vi "Test.vi"() -> ()   [LabVIEW 2015, in "Database.lvclass"]
uses:
  Database.lvclass
  <vilib>/addons/database/Auxilliary.llb/DB Tools Column Info.ctl
  <vilib>/addons/database/Auxilliary.llb/DB Tools DataTypes.ctl
  <vilib>/addons/database/NI_Database_API.lvlib
panel:
  out "Not Empty":bool
  out "eof?":bool
  in  "data":T1
  in  "columns":string[](array[string])
  out "recordset data":variant[][](array[variant])
  in  "condition":string
  in  "column information":T2[](array[typedef])
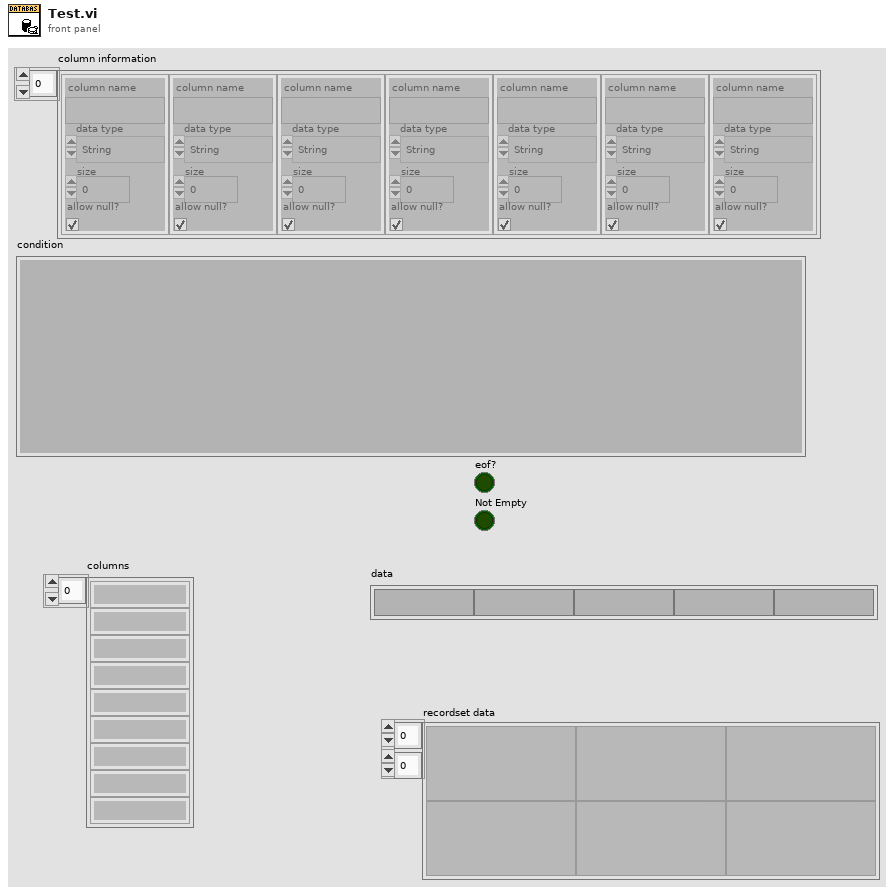
[diagram p1: front panel]
types:
  T1 = cluster{"String":string, "String 2":string, "String 3":string, "String 4":string, "String 5":string}
  T2 = typedef "NI_Database_API.lvlib/DB Tools Column Info.ctl" = cluster{"column name":string, "data type":T3, "size":i32, "allow null?":bool}
  T3 = typedef "NI_Database_API.lvlib/DB Tools DataTypes.ctl" = enum16{"String", "Long (I32)", "Single (SGL)", "Double (DBL)", "Date/Time", "Binary"}
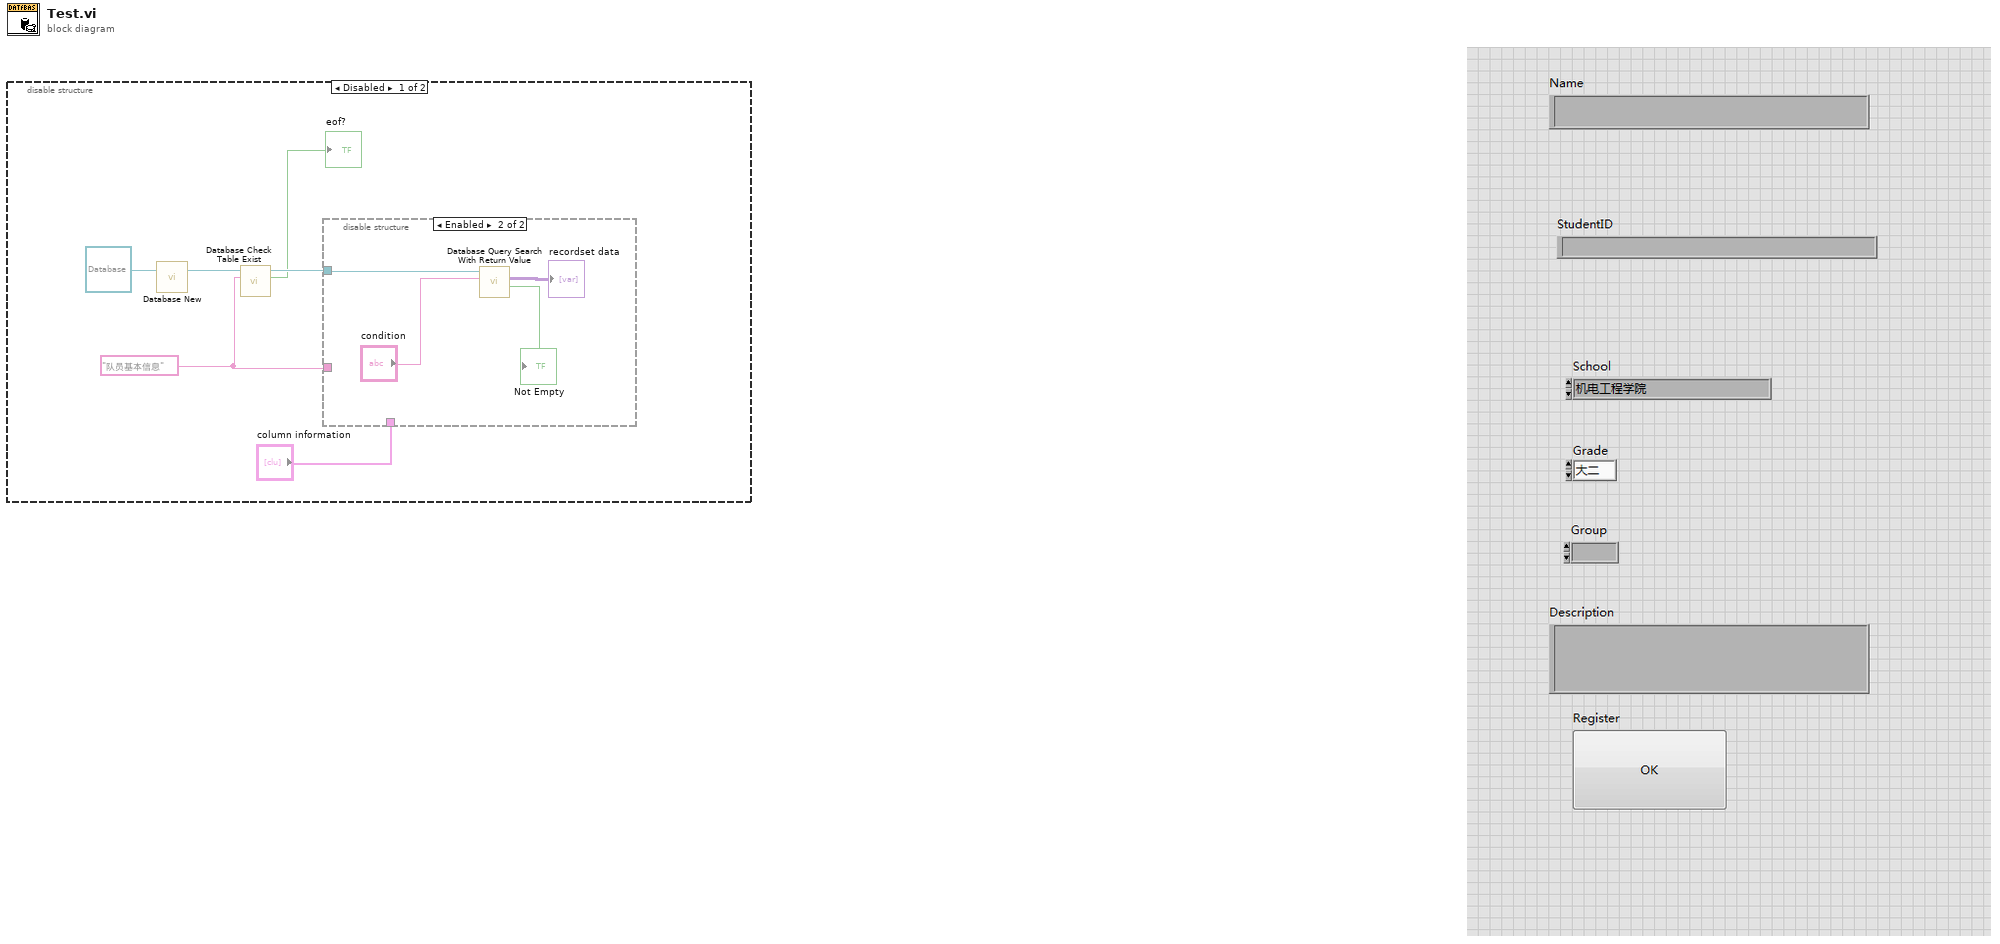
[diagram p0: block diagram]
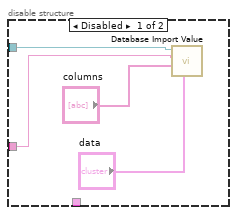
[diagram p2: hidden frame]
diagram:
  n1 = disable-structure shown="Disabled" {
    frame Disabled {
      w2 = "队员基本信息" ("table")
      n2 = call "Database New.vi"("object in"=refnum<class "Database.lvclass"> refnum ("Database.lvlib:Database")) -> ("object out"=w4:refnum<class "Database.lvclass">)  [unwired: 1 in, 1 out]
      n3 = call "Database Check Table Exist.vi"("Table"=w2, "Database in"=w4) -> ("Exit?"=→"eof?":bool, "Database out"=w3:refnum<class "Database.lvclass">)  [unwired: 7 in, 1 out]
      n4 = disable-structure shown="Enabled" {
        disable-tunnel: w3 -> [w10 w14]
        disable-tunnel: w2 -> [w9 _]
        disable-tunnel: "column information" -> [_ _]
        frame Disabled {
          n5 = call "Database Import Value.vi"("data"="data", "columns"="columns", "table"=w9, "object in"=w10) -> ()  [unwired: 6 in, 2 out]
        }
        frame Enabled {
          n6 = call "Database Query Search With Return Value.vi"("SQL query"="condition", "object in"=w14) -> ("Not Empty"=→"Not Empty":bool, "recordset data"=→"recordset data":variant[][])  [unwired: 6 in, 2 out]
        }
      }
    }
    frame Enabled {
    }
  }
